vi "workers2.vi"(0 "queue DS18B20":refnum<queue>, 1 "queue BMP180":refnum<queue>, 2 "queue potentiometer":refnum<queue>, 3 "queue ACS712-30A":refnum<queue>, 4 "result queue":refnum<queue>, 5 "HTTP client handle":T1) -> (14 "result queue out":refnum<queue>, 15 "result queue error out":errorcluster, 18 "client handle out":T1, 19 "client handle error out":errorcluster)   [LabVIEW 2016]
uses:
  <vilib>/httpClient/ClientHandle.ctl
  <vilib>/Utility/error.llb/DialogType.ctl
  <vilib>/gmath/NI_Gmath.lvlib
  <vilib>/httpClient/LabVIEWHTTPClient.lvlib
panel:
  out "sorted array":cluster{string, dbl}[](array[cluster])
  out "unsorted elements":cluster{string, dbl}[](array[cluster])
  out "request":string
  out "# elements in ACS712-30A queue":i32
  out "# elements inpotentiometer  queue":i32
  out "# elements in DS18B20 queue":i32
  out "# elements in BMP180 queue":i32
  out "error out":errorcluster
  out "headers":string
  out "body":string
  out "remaining elements 4":dbl[](array[numeric])
  out "remaining elements 3":dbl[](array[numeric])
  out "remaining elements 2":dbl[](array[numeric])
  out "remaining elements":dbl[](array[numeric])
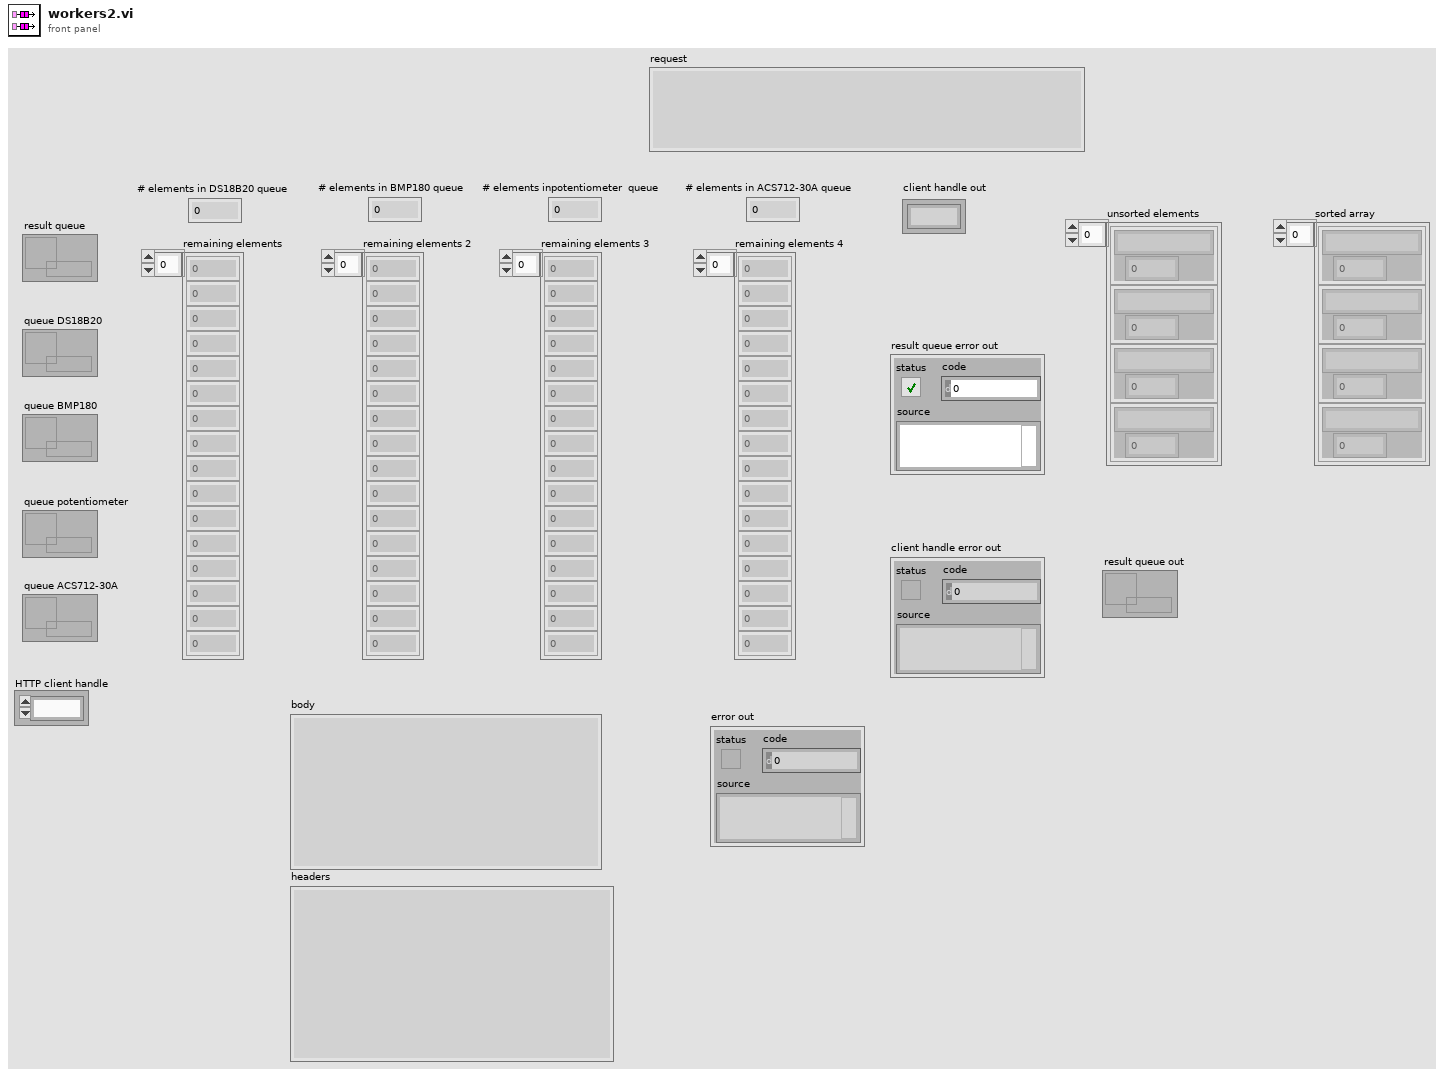
[diagram p1: front panel]
types:
  T1 = typedef "LabVIEWHTTPClient.lvlib/ClientHandle.ctl" = refnum<k1>
  T2 = enum16{"arithmetic", "geometric", "harmonic", "trimmed", "median"}
  T3 = typedef "DialogType.ctl" = u16
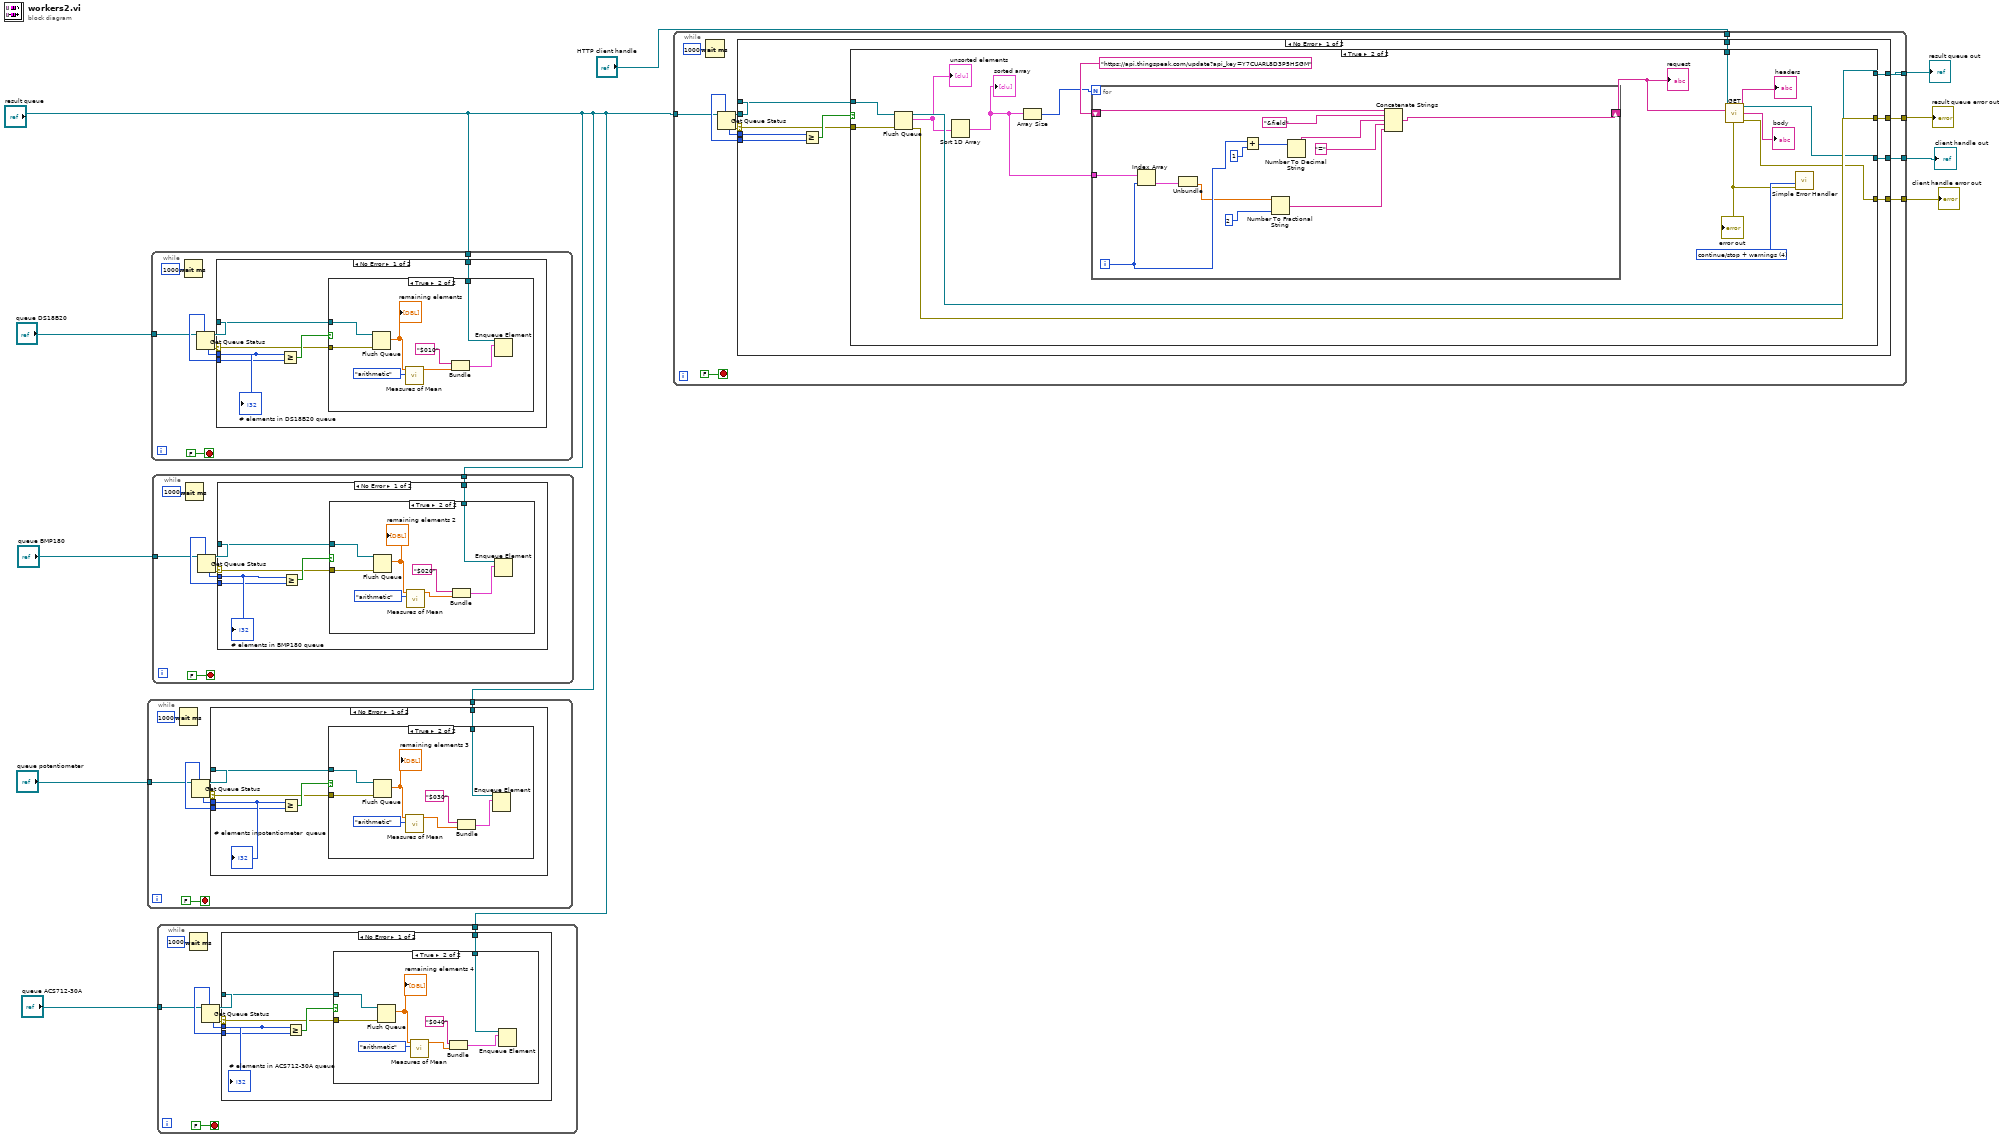
[diagram p0: block diagram]
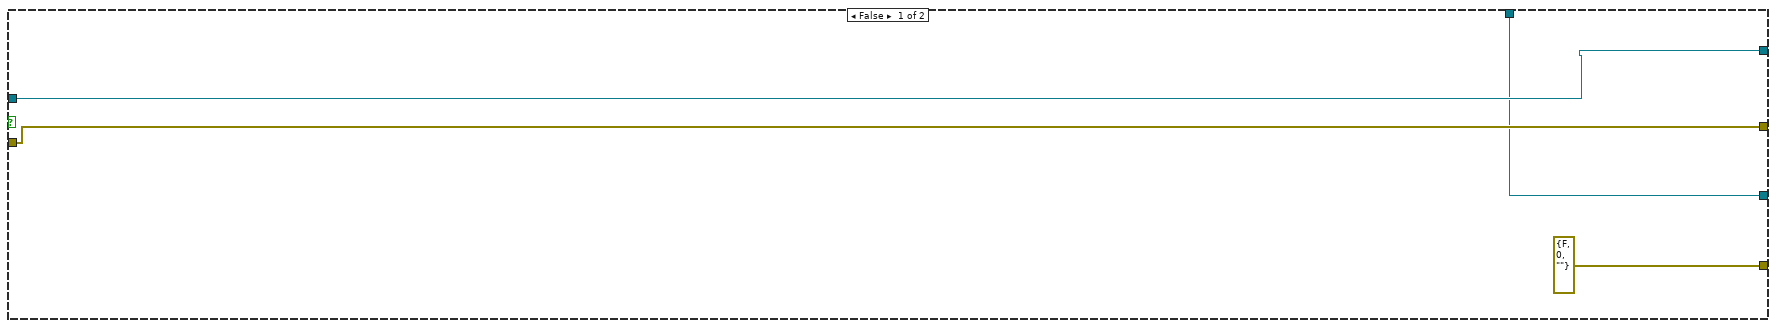
[diagram p2: hidden frame]
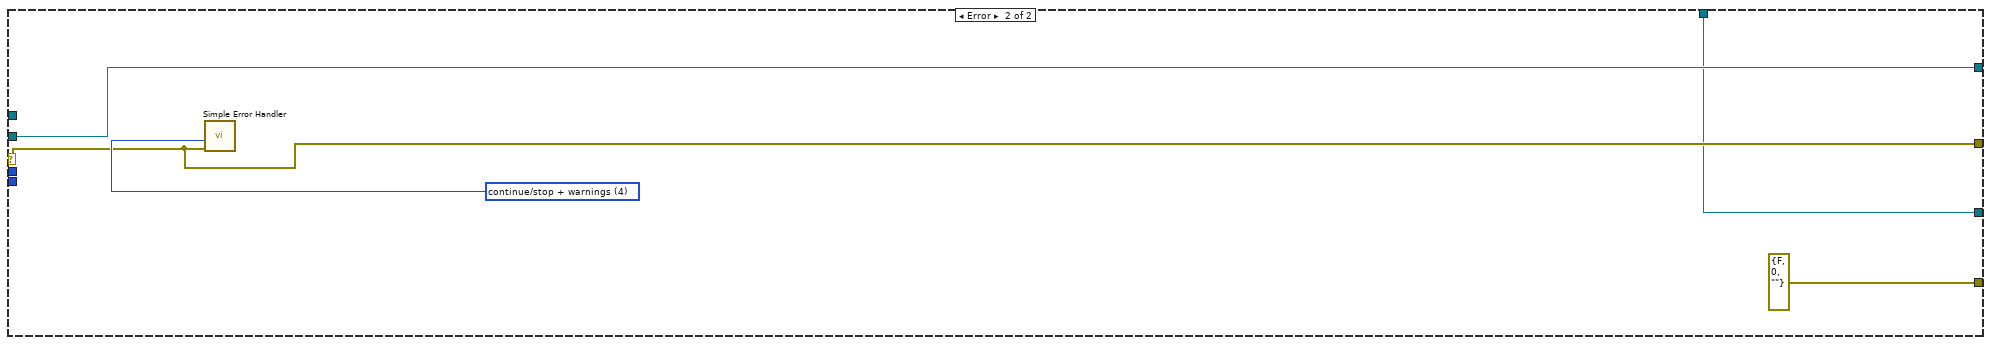
[diagram p3: hidden frame]
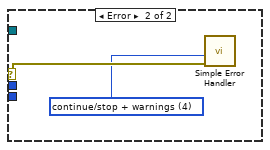
[diagram p5: hidden frame]
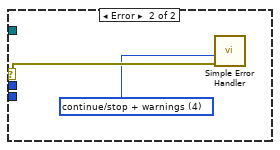
[diagram p7: hidden frame]
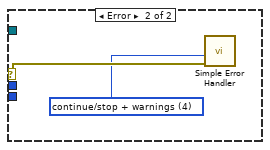
[diagram p9: hidden frame]
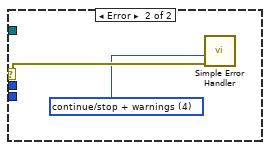
[diagram p11: hidden frame]
diagram:
  n1 = while {
    tunnel: "queue potentiometer" -> [w12]
    tunnel: "result queue" -> [w11]
    stop <- FALSE stop-if-true
    n2 = Wait (ms)(milliseconds to wait=u32 1000) -> ()  [unwired: 1 out]
    n3 = Get Queue Status(queue=w12) -> (queue out=w13:refnum<queue>, max queue size=w14:i32, error out=w16:errorcluster, # elements in queue=w15:i32)  [unwired: 2 in, 4 out]
    n4 = case shown="No Error" w16 {
      selector: w16 -> [w21 w34]
      tunnel: w15 -> [w23 _]
      tunnel: w14 -> [w22 _]
      tunnel: w13 -> [w20 _]
      tunnel: w11 -> [w19 _]
      frame No Error {
        n5 = Greater Or Equal?(x=w23, y=w22) -> (x >= y?=w24:bool)
        n6 = case shown="True" w24 {
          tunnel: w21 -> [_ w32]
          tunnel: w20 -> [_ w31]
          tunnel: w19 -> [_ w28]
          frame False {
          }
          frame True {
            n7 = Flush Queue(queue=w31, error in (no error)=w32) -> (remaining elements=w30:dbl[])  [unwired: 2 out]
            "remaining elements 3" <- w30
            n8 = call <vilib>:"Measures of Mean.vi"("type"=T2."arithmetic", "x array"=w30) -> ("mean value"=w27:dbl)  [unwired: 8 in, 1 out]
            n9 = Bundle("$030", "mean value"=w27) -> (w26:cluster{string, "mean value":dbl})  [unwired: 1 in]
            n10 = Enqueue Element(queue=w28, element=w26) -> ()  [unwired: 2 in, 3 out]
          }
        }
        "# elements inpotentiometer  queue" <- w23
      }
      frame Error {
        w33 = T3 4 items=["no dialog", "OK message", "continue or stop message", "OK message + warnings", "continue/stop + warnings"] ("type of dialog (OK msg:1)")
        n11 = call <vilib>:"Simple Error Handler.vi"("type of dialog (OK msg:1)"=w33, "error in (no error)"=w34) -> ()  [unwired: 3 in, 5 out]
      }
    }
  }
  n12 = while {
    tunnel: "queue DS18B20" -> [w36]
    tunnel: "result queue" -> [w35]
    stop <- FALSE stop-if-true
    n13 = Wait (ms)(milliseconds to wait=u32 1000) -> ()  [unwired: 1 out]
    n14 = Get Queue Status(queue=w36) -> (queue out=w37:refnum<queue>, max queue size=w38:i32, error out=w40:errorcluster, # elements in queue=w39:i32)  [unwired: 2 in, 4 out]
    n15 = case shown="No Error" w40 {
      selector: w40 -> [w45 w58]
      tunnel: w39 -> [w47 _]
      tunnel: w38 -> [w46 _]
      tunnel: w37 -> [w44 _]
      tunnel: w35 -> [w43 _]
      frame No Error {
        n16 = Greater Or Equal?(x=w47, y=w46) -> (x >= y?=w48:bool)
        n17 = case shown="True" w48 {
          tunnel: w45 -> [_ w56]
          tunnel: w44 -> [_ w55]
          tunnel: w43 -> [_ w52]
          frame False {
          }
          frame True {
            n18 = Flush Queue(queue=w55, error in (no error)=w56) -> (remaining elements=w54:dbl[])  [unwired: 2 out]
            "remaining elements" <- w54
            n19 = call <vilib>:"Measures of Mean.vi"("type"=T2."arithmetic", "x array"=w54) -> ("mean value"=w51:dbl)  [unwired: 8 in, 1 out]
            n20 = Bundle("$010", "mean value"=w51) -> (w49:cluster{string, "mean value":dbl})  [unwired: 1 in]
            n21 = Enqueue Element(queue=w52, element=w49) -> ()  [unwired: 2 in, 3 out]
          }
        }
        "# elements in DS18B20 queue" <- w47
      }
      frame Error {
        w57 = T3 4 items=["no dialog", "OK message", "continue or stop message", "OK message + warnings", "continue/stop + warnings"] ("type of dialog (OK msg:1)")
        n22 = call <vilib>:"Simple Error Handler.vi"("type of dialog (OK msg:1)"=w57, "error in (no error)"=w58) -> ()  [unwired: 3 in, 5 out]
      }
    }
  }
  n23 = while {
    tunnel: "queue BMP180" -> [w60]
    tunnel: "result queue" -> [w59]
    stop <- FALSE stop-if-true
    n24 = Wait (ms)(milliseconds to wait=u32 1000) -> ()  [unwired: 1 out]
    n25 = Get Queue Status(queue=w60) -> (queue out=w61:refnum<queue>, max queue size=w62:i32, error out=w64:errorcluster, # elements in queue=w63:i32)  [unwired: 2 in, 4 out]
    n26 = case shown="No Error" w64 {
      selector: w64 -> [w69 w82]
      tunnel: w63 -> [w71 _]
      tunnel: w62 -> [w70 _]
      tunnel: w61 -> [w68 _]
      tunnel: w59 -> [w67 _]
      frame No Error {
        n27 = Greater Or Equal?(x=w71, y=w70) -> (x >= y?=w72:bool)
        n28 = case shown="True" w72 {
          tunnel: w69 -> [_ w80]
          tunnel: w68 -> [_ w79]
          tunnel: w67 -> [_ w76]
          frame False {
          }
          frame True {
            n29 = Flush Queue(queue=w79, error in (no error)=w80) -> (remaining elements=w78:dbl[])  [unwired: 2 out]
            "remaining elements 2" <- w78
            n30 = call <vilib>:"Measures of Mean.vi"("type"=T2."arithmetic", "x array"=w78) -> ("mean value"=w74:dbl)  [unwired: 8 in, 1 out]
            n31 = Bundle("$020", "mean value"=w74) -> (w75:cluster{string, "mean value":dbl})  [unwired: 1 in]
            n32 = Enqueue Element(queue=w76, element=w75) -> ()  [unwired: 2 in, 3 out]
          }
        }
        "# elements in BMP180 queue" <- w71
      }
      frame Error {
        w81 = T3 4 items=["no dialog", "OK message", "continue or stop message", "OK message + warnings", "continue/stop + warnings"] ("type of dialog (OK msg:1)")
        n33 = call <vilib>:"Simple Error Handler.vi"("type of dialog (OK msg:1)"=w81, "error in (no error)"=w82) -> ()  [unwired: 3 in, 5 out]
      }
    }
  }
  n34 = while {
    tunnel: "queue ACS712-30A" -> [w84]
    tunnel: "result queue" -> [w83]
    stop <- FALSE stop-if-true
    n35 = Wait (ms)(milliseconds to wait=u32 1000) -> ()  [unwired: 1 out]
    n36 = Get Queue Status(queue=w84) -> (queue out=w85:refnum<queue>, max queue size=w86:i32, error out=w88:errorcluster, # elements in queue=w87:i32)  [unwired: 2 in, 4 out]
    n37 = case shown="No Error" w88 {
      selector: w88 -> [w93 w106]
      tunnel: w87 -> [w95 _]
      tunnel: w86 -> [w94 _]
      tunnel: w85 -> [w92 _]
      tunnel: w83 -> [w91 _]
      frame No Error {
        n38 = Greater Or Equal?(x=w95, y=w94) -> (x >= y?=w96:bool)
        n39 = case shown="True" w96 {
          tunnel: w93 -> [_ w104]
          tunnel: w92 -> [_ w103]
          tunnel: w91 -> [_ w100]
          frame False {
          }
          frame True {
            n40 = Flush Queue(queue=w103, error in (no error)=w104) -> (remaining elements=w102:dbl[])  [unwired: 2 out]
            "remaining elements 4" <- w102
            n41 = call <vilib>:"Measures of Mean.vi"("type"=T2."arithmetic", "x array"=w102) -> ("mean value"=w98:dbl)  [unwired: 8 in, 1 out]
            n42 = Bundle("$040", "mean value"=w98) -> (w99:cluster{string, "mean value":dbl})  [unwired: 1 in]
            n43 = Enqueue Element(queue=w100, element=w99) -> ()  [unwired: 2 in, 3 out]
          }
        }
        "# elements in ACS712-30A queue" <- w95
      }
      frame Error {
        w105 = T3 4 items=["no dialog", "OK message", "continue or stop message", "OK message + warnings", "continue/stop + warnings"] ("type of dialog (OK msg:1)")
        n44 = call <vilib>:"Simple Error Handler.vi"("type of dialog (OK msg:1)"=w105, "error in (no error)"=w106) -> ()  [unwired: 3 in, 5 out]
      }
    }
  }
  n45 = while {
    tunnel: "result queue" -> [w114]
    tunnel: "HTTP client handle" -> [w112]
    tunnel: [w111] -> w5
    tunnel: [w110] -> w1
    tunnel: [w108] -> w4
    tunnel: [w107] -> w3
    stop <- FALSE stop-if-true
    n46 = Wait (ms)(milliseconds to wait=u32 1000) -> ()  [unwired: 1 out]
    n47 = Get Queue Status(queue=w114) -> (queue out=w109:refnum<queue>, max queue size=w115:i32, error out=w116:errorcluster, # elements in queue=w113:i32)  [unwired: 2 in, 4 out]
    n48 = case shown="No Error" w116 {
      selector: w116 -> [w126 w163]
      tunnel: w115 -> [w127 _]
      tunnel: w109 -> [w125 _]
      tunnel: w113 -> [w124 _]
      tunnel: w112 -> [w123 w161]
      tunnel: [w122 w163] -> w111
      tunnel: [w121 w164] -> w110
      tunnel: w109 -> [_ w164]
      tunnel: [w120 w161] -> w108
      tunnel: [w119 errorcluster {"status"=FALSE, "code"=0, "source"=""} ("error out")] -> w107
      frame No Error {
        n49 = Greater Or Equal?(x=w124, y=w127) -> (x >= y?=w128:bool)
        n50 = case shown="True" w128 {
          tunnel: w126 -> [w132 w147]
          tunnel: w125 -> [w131 w146]
          tunnel: w123 -> [w130 w145]
          tunnel: [w132 w142] -> w122
          tunnel: [w131 w141] -> w121
          tunnel: [w130 w139] -> w120
          tunnel: [errorcluster {"status"=FALSE, "code"=0, "source"=""} ("error out") w138] -> w119
          frame False {
          }
          frame True {
            w140 = T3 4 items=["no dialog", "OK message", "continue or stop message", "OK message + warnings", "continue/stop + warnings"] ("type of dialog (OK msg:1)")
            n51 = Flush Queue(queue=w146, error in (no error)=w147) -> (queue out=w141:refnum<queue>, remaining elements=w137:cluster{string, dbl}[], error out=w142:errorcluster)
            "unsorted elements" <- w137
            n52 = Sort 1D Array(array=w137) -> (sorted array=w134:cluster{string, dbl}[])
            "sorted array" <- w134
            n53 = Array Size(array=w134) -> (size(s)=w135:i32)
            n54 = for {
              N: w135 -> [_]
              shift-right: [w152] -> w133
              shift-left: "https://api.thingspeak.com/update?api_key=Y7CUARL8D3P5HSGM" -> [w157]
              tunnel: w134 -> [w151]
              i -> [w150]
              n55 = Index Array(array=w151, index=w150) -> (element=w149:cluster{string, dbl})
              n56 = Unbundle(w149) -> (w148:dbl)  [unwired: 1 out]
              n57 = Add(x=w150, y=1) -> (x+y=w158:i32)
              n58 = Number To Fractional String(number=w148, precision (6)=i16 2) -> (F-format string=w153:string)  [unwired: 2 in]
              n59 = Number To Decimal String(number=w158) -> (decimal integer string=w155:string)  [unwired: 1 in]
              n60 = Concatenate Strings(w157, "&field", w155, "=", w153) -> (w152:string)
            }
            "request" <- w133
            n61 = call <vilib>:"GET.vi"("client handle"=w145, "url"=w133) -> ("client handle out"=w139:T1, "headers"=→"headers":string, "body"=→"body":string, "error out"=w138:errorcluster)  [unwired: 10 in]
            "error out" <- w138
            n62 = call <vilib>:"Simple Error Handler.vi"("type of dialog (OK msg:1)"=w140, "error in (no error)"=w138) -> ()  [unwired: 3 in, 5 out]
          }
        }
      }
      frame Error {
        w165 = T3 4 items=["no dialog", "OK message", "continue or stop message", "OK message + warnings", "continue/stop + warnings"] ("type of dialog (OK msg:1)")
        n63 = call <vilib>:"Simple Error Handler.vi"("type of dialog (OK msg:1)"=w165, "error in (no error)"=w163) -> ()  [unwired: 3 in, 5 out]
      }
    }
  }
  "result queue error out" <- w5
  "client handle out" <- w4
  "client handle error out" <- w3
  "result queue out" <- w1
